vi "run_ACLooper.vi"() -> ()   [LabVIEW 2015]
uses:
  <vilib>/Platform/TimedLoop/XDataNode/timing_clust.ctl
  <vilib>/Platform/TimedLoop/XDataNode/nitl_modes.ctl
  <vilib>/Platform/TimedLoop/XDataNode/wakeup.ctl
  <vilib>/measure/matone.llb/Extract Multiple Tone Information 1 Chan.vi
  <vilib>/measure/maspectr.llb/FFT Spectrum (Mag-Phase) for 1 Chan.vi
  <vilib>/measure/matone.llb/Extract Single Tone Information 1 Chan.vi
  <vilib>/Utility/file.llb/Write To Spreadsheet File (string).vi
  <vilib>/Platform/TimedLoop/XDataNode/XDataNode.xnode
  <vilib>/Platform/TimedLoop/XDataNode/XDNodeRunTimeDep.lvlib
  <vilib>/measure/NI_MAPro.lvlib
  <vilib>/ptbypt/NI_PtbyPt.lvlib
panel:
  in  "?":T1(tab)
  in  "Number of Channel":string(combo)="2"
  in  "Volume of Sample (ml)":dbl=0.498
  in  "Concentration of Sample (mg/ml)":dbl=1.19
  in  "Select Serial Port":refnum<visa-resource-name>="COM6"
  in  "Temperature \nMeasurement":bool
  out "Value Ch4":dbl format="%.2f"
  out "Value Ch3":dbl format="%.2f"
  out "Status Ch4":bool
  out "Status Ch3":bool
  out "Status Ch2":bool
  out "Status Ch1":bool
  out "Unit Ch 4":string=" "
  out "Unit Ch 3":string=" "
  out "Value Ch2":dbl format="%.2f"
  out "Unit Ch2":string=" "
  out "Unit Ch1":string=" "
  out "Value Ch1":dbl format="%.2f"
  out "Temperature Streaming":T2(graph)={"Value_1"=28.19, "Value_2"=24.43, "Value_3"=0.0, "Value_4"=0.0}
  in  "Clear the Figure":bool
  in  "Stop":bool
  in  "Start":bool
  in  "Graph ChA":bool=TRUE
  out "Channel A":i16[](graph)
  in  "Enable ChA":bool=TRUE
  in  "Channel A Settings":T3={"Enabled"=TRUE, "DC Coupled"=TRUE, "Range"=6} {"Range" items=["10 mV", "20 mV", "50 mV", "100 mV", "200 mV", "500 mV", "1 V", "2 V", "5 V", "10 V", "20 V", "50 V ", "100 V"]}
  out "Numeric":i32
  in  "stop":bool
  in  "PicoScope":bool=TRUE
  out "Frequency Interpolate / Hz A":dbl format="%#_8g"
  out "H (A/m) / Vpp":dbl
  in  "ChA sample length":i32=5
  in  "H sample length":i32=5
  in  "Filter H":bool=TRUE
  in  "Rokoski (V(mV)/I(A))":dbl=20.0
  in  "Turns of Coil":dbl=6.0
  out "Current (A)":dbl
  in  "Filter ChA":bool=TRUE
  in  "H calculator":bool=TRUE
  out "H / Vpp":cluster{dbl}(graph)
  out "Vpp A":dbl
  out "Frequency Tracking A":cluster{"Frequency Interpolate / Hz":dbl}(graph)
  in  "Balance":bool
  in  "Description":string="no sample"
  in  "Filename":string="\\Oct04_warmup_2ch_18_4V.txt"
  in  "Time Target (min)":dbl=600.0 format="%#_13g"
  out "Measurement Complete":bool caption="Time has Elapsed"
  out "Remaining  time":dbl format="%<%H:%M:%S>t"
  in  "Record":bool
  in  "File Path":path=path "C:/Users/Fangyu/Google Drive/3_UCL MRes Medical Device/M0_Individual Project/A008 Experiments/C004_LabViewPicoScope/MACH/data"
  in  "Recording Period (ms)":i64=1000
  out "Phase (deg)":dbl format="%.2p"
  in  "MACH:":string(combo)="1. MACH/HBL Invitro 6Turn"
  out "PicoScope V range":dbl
  out "Recording Time":dbl format="%<%H:%M:%S>t"
  in  "Channel B Settings":T3={"Enabled"=TRUE, "DC Coupled"=TRUE, "Range"=7} {"Range" items=["10 mV", "20 mV", "50 mV", "100 mV", "200 mV", "500 mV", "1 V", "2 V", "5 V", "10 V", "20 V", "50 V ", "100 V"]}
  in  "Enable ChB":bool
  out "Channel B":i16[](graph)
  in  "Acquisition Settings":T4={"preTriggerSamples"=0, "postTriggerSamples"=20000, "timebase"=2, "Aggregate Data"=FALSE, "Down Sample Ratio"=1, "Four Channel Device"=FALSE, "Oversample"=1} {"Down Sample Ratio" min=1 step=1}
  in  "Sampling Frequency":dbl=250000000.0
  in  "Trigger Settings":T5={"Trigger Enabled"=TRUE, "Trigger Source"=enum."Channel A", "Trigger Threshold (16-bit counts)"=100, "Trigger Direction"=3, "Trigger Delay (samples)"=20, "Auto Trigger Time (ms)"=0} {"Trigger Direction" items=["Rising"=2, "Falling"=3]}
  in  "History data for graph reset":cluster{dbl}[](array[cluster])
  in  "Calibration":bool
  in  "Commands":string
  in  "Send/Enter:":bool
  in  "Slect Probet Channel":string="1,3"
  in  "Send/Enter: 2":bool
  in  "Reset":bool
  in  "Check Param":bool
  out "read buffer":string="PS??\r\nPS??\r\nAE??\r\n\n <ignored>\r\nPS=1,2\r\n"
  out "error out 2":errorcluster={"status"=TRUE, "code"=-1073807339, "source"="VISA Read in Test1.vi"}
  # "Setting of Luxtron Thermometer"
  # "1.  Enter Cal Temperature in 'Commands' above\n     (CT=XX.X)  and press 'Send' button\n2.  Press button below\n3.  Calibration may take ~ 1 min."
  # "The content of recorded data:\n1st Row; 2nd Row; 3rd Row; 4th Row; 5th Row; 6th Row; 7th Row; 8th Row; 9th Row\nTime; Field Strength; Frequency; Value Ch1; Value Ch2; Value Ch3; Value Ch4; Maximal Frequency; ;Frequency Drop"
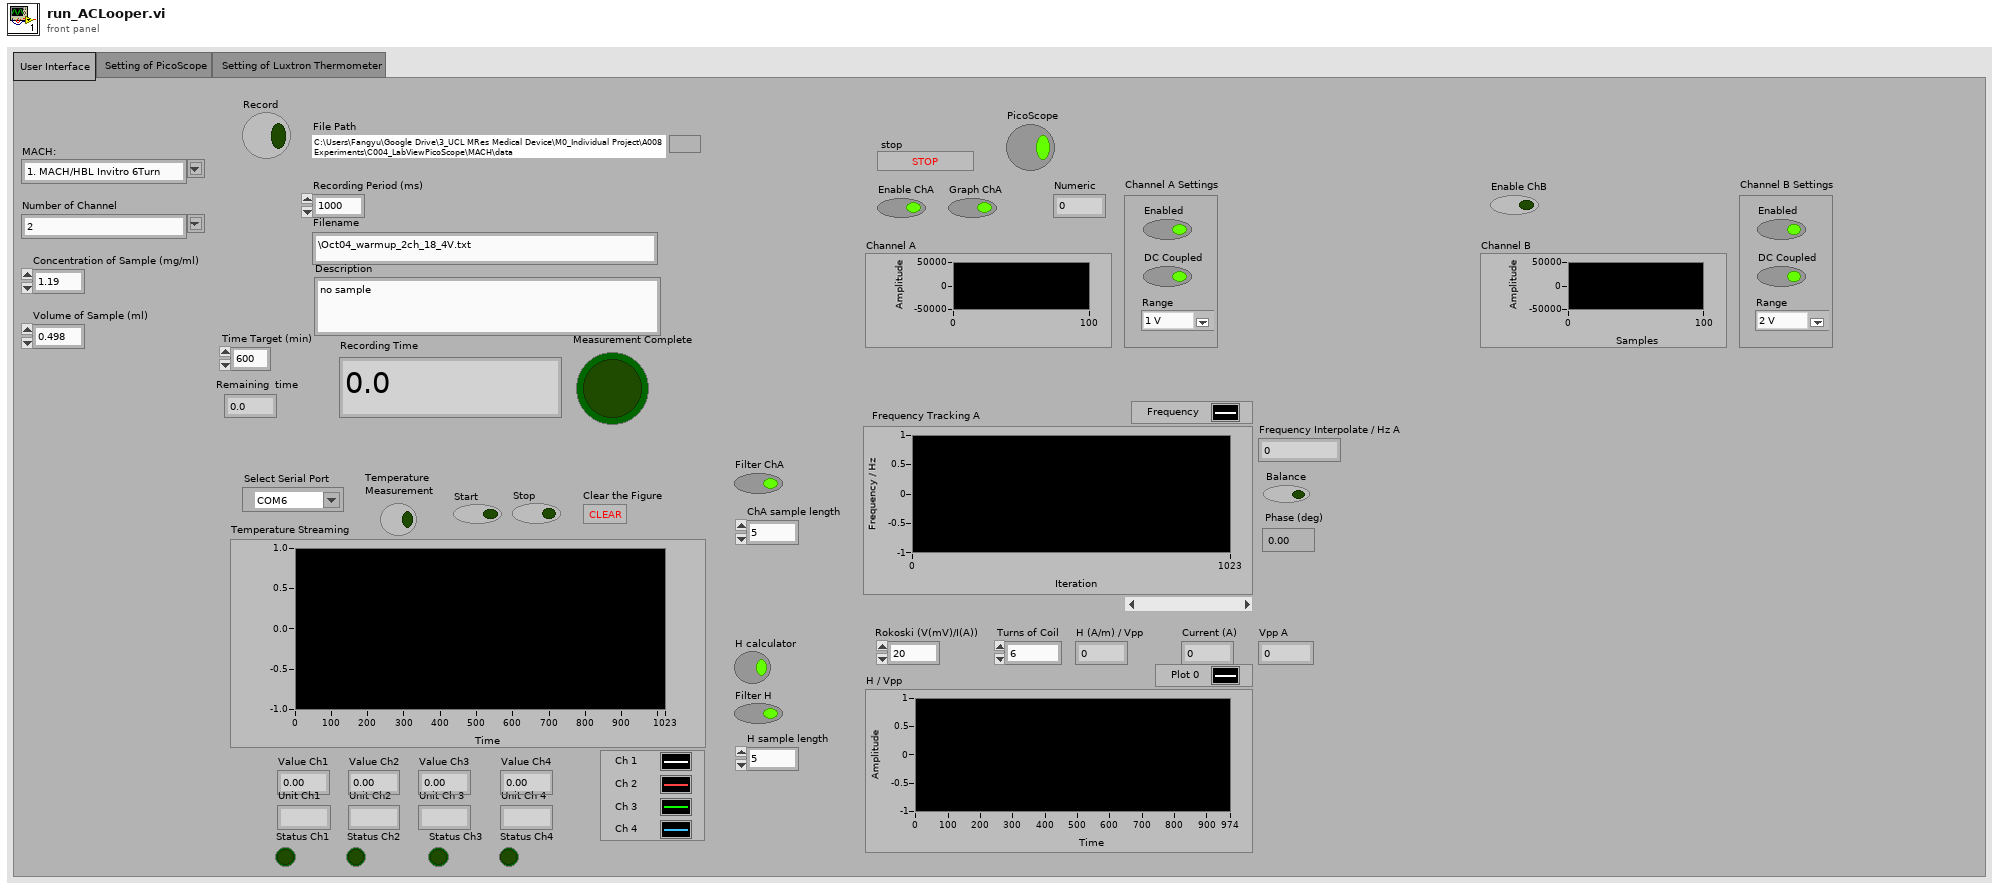
[diagram p1: front panel]
types:
  T1 = enum32{"User Interface", " Setting of PicoScope", " Setting of Luxtron Thermometer"}
  T2 = cluster{"Value_1":dbl, "Value_2":dbl, "Value_3":dbl, "Value_4":dbl}
  T3 = cluster{"Enabled":bool, "DC Coupled":bool, "Range":u16}
  T4 = cluster{"preTriggerSamples":i32, "postTriggerSamples":i32, "timebase":u32, "Aggregate Data":bool, "Down Sample Ratio":u32, "Four Channel Device":bool, "Oversample":i16}
  T5 = cluster{"Trigger Enabled":bool, "Trigger Source":enum16{"Channel A", "Channel B", "Channel C", "Channel D"}, "Trigger Threshold (16-bit counts)":i16, "Trigger Direction":u16, "Trigger Delay (samples)":u32, "Auto Trigger Time (ms)":i16}
  T6 = cluster{"Status_1":bool, "Value_1":dbl, "Unit_1":string, "Status_2":bool, "Value_2":dbl, "Unit_2":string, "Status_3":bool, "Value_3":dbl, "Unit_3":string, "Status_4":bool, "Value_4":dbl, "Unit_4":string}
  T7 = enum32{"none", "input signal", "detected signal", "residual signal"}
  T8 = cluster{"Peak-to-Peak Voltage (microvolts)":u32, "Offset Voltage (microvolts)":i32, "Wave Type":i16, "Sweep Type":i32, "Shots":u32, "Sweeps":u32, "Trigger Type":i32, "Trigger Source":i32, "Ext. Threshold (ADC count)":i16, "White Noise":bool}
  T9 = cluster{"Channel D Buffer":i16[], "Channel C Buffer":i16[], "Channel B Buffer":i16[], "Channel A Buffer":i16[]}
  T10 = cluster{"detected frequency":dbl, "detected amplitude":dbl, "detected phase (deg)":dbl}[]
  T11 = cluster{"magnitude[0]":dbl, "magnitude[1]":dbl, "magnitude[2]":dbl, "magnitude[3]":dbl, "magnitude[4]":dbl, "magnitude[5]":dbl, "magnitude[6]":dbl, "magnitude[7]":dbl, "magnitude[8]":dbl}
  T12 = typedef "XDNodeRunTimeDep.lvlib/timing_clust.ctl" = cluster{"Expected End [f-1]":u64, "Actual End [f-1]":u64, "Finished Late? [f-1]":bool, "Expected End [i-1]":u64, "Actual End [i-1]":u64, "Finished Late? [i-1]":bool, "Expected Start [i]":u64, "Actual Start [i]":u64, "Expected Start [f]":u64, "Actual Start [f]":u64, "Source Name":string, "Structure Name":string, "Period":i64, "Deadline":i64, "Offset":i64, "Start":i64, "Priority":i32, "Timeout":i32, "Mode":T13, "Wakeup Reason":T14, "Error":errorcluster, "Source Type":string, "Secondary Source Type":string, "Global End Time":u64, "Global Start Time":u64, "Frame Duration":u64, "Iteration Duration":u64, "Assigned CPU":i32, "I/O Scan Engine Mode":u32}
  T13 = typedef "XDNodeRunTimeDep.lvlib/nitl_modes.ctl" = enum32{"No Change", "Process missed periods, maintain original phase", "Discard missed periods, maintain original phase", "Process missed periods, ignore original phase", "Discard missed periods, ignore original phase"}
  T14 = typedef "XDNodeRunTimeDep.lvlib/wakeup.ctl" = enum32{"Normal", "Aborted", "Asynchronous wakeup", "Timing source error", "Timed loop error", "Timeout"}
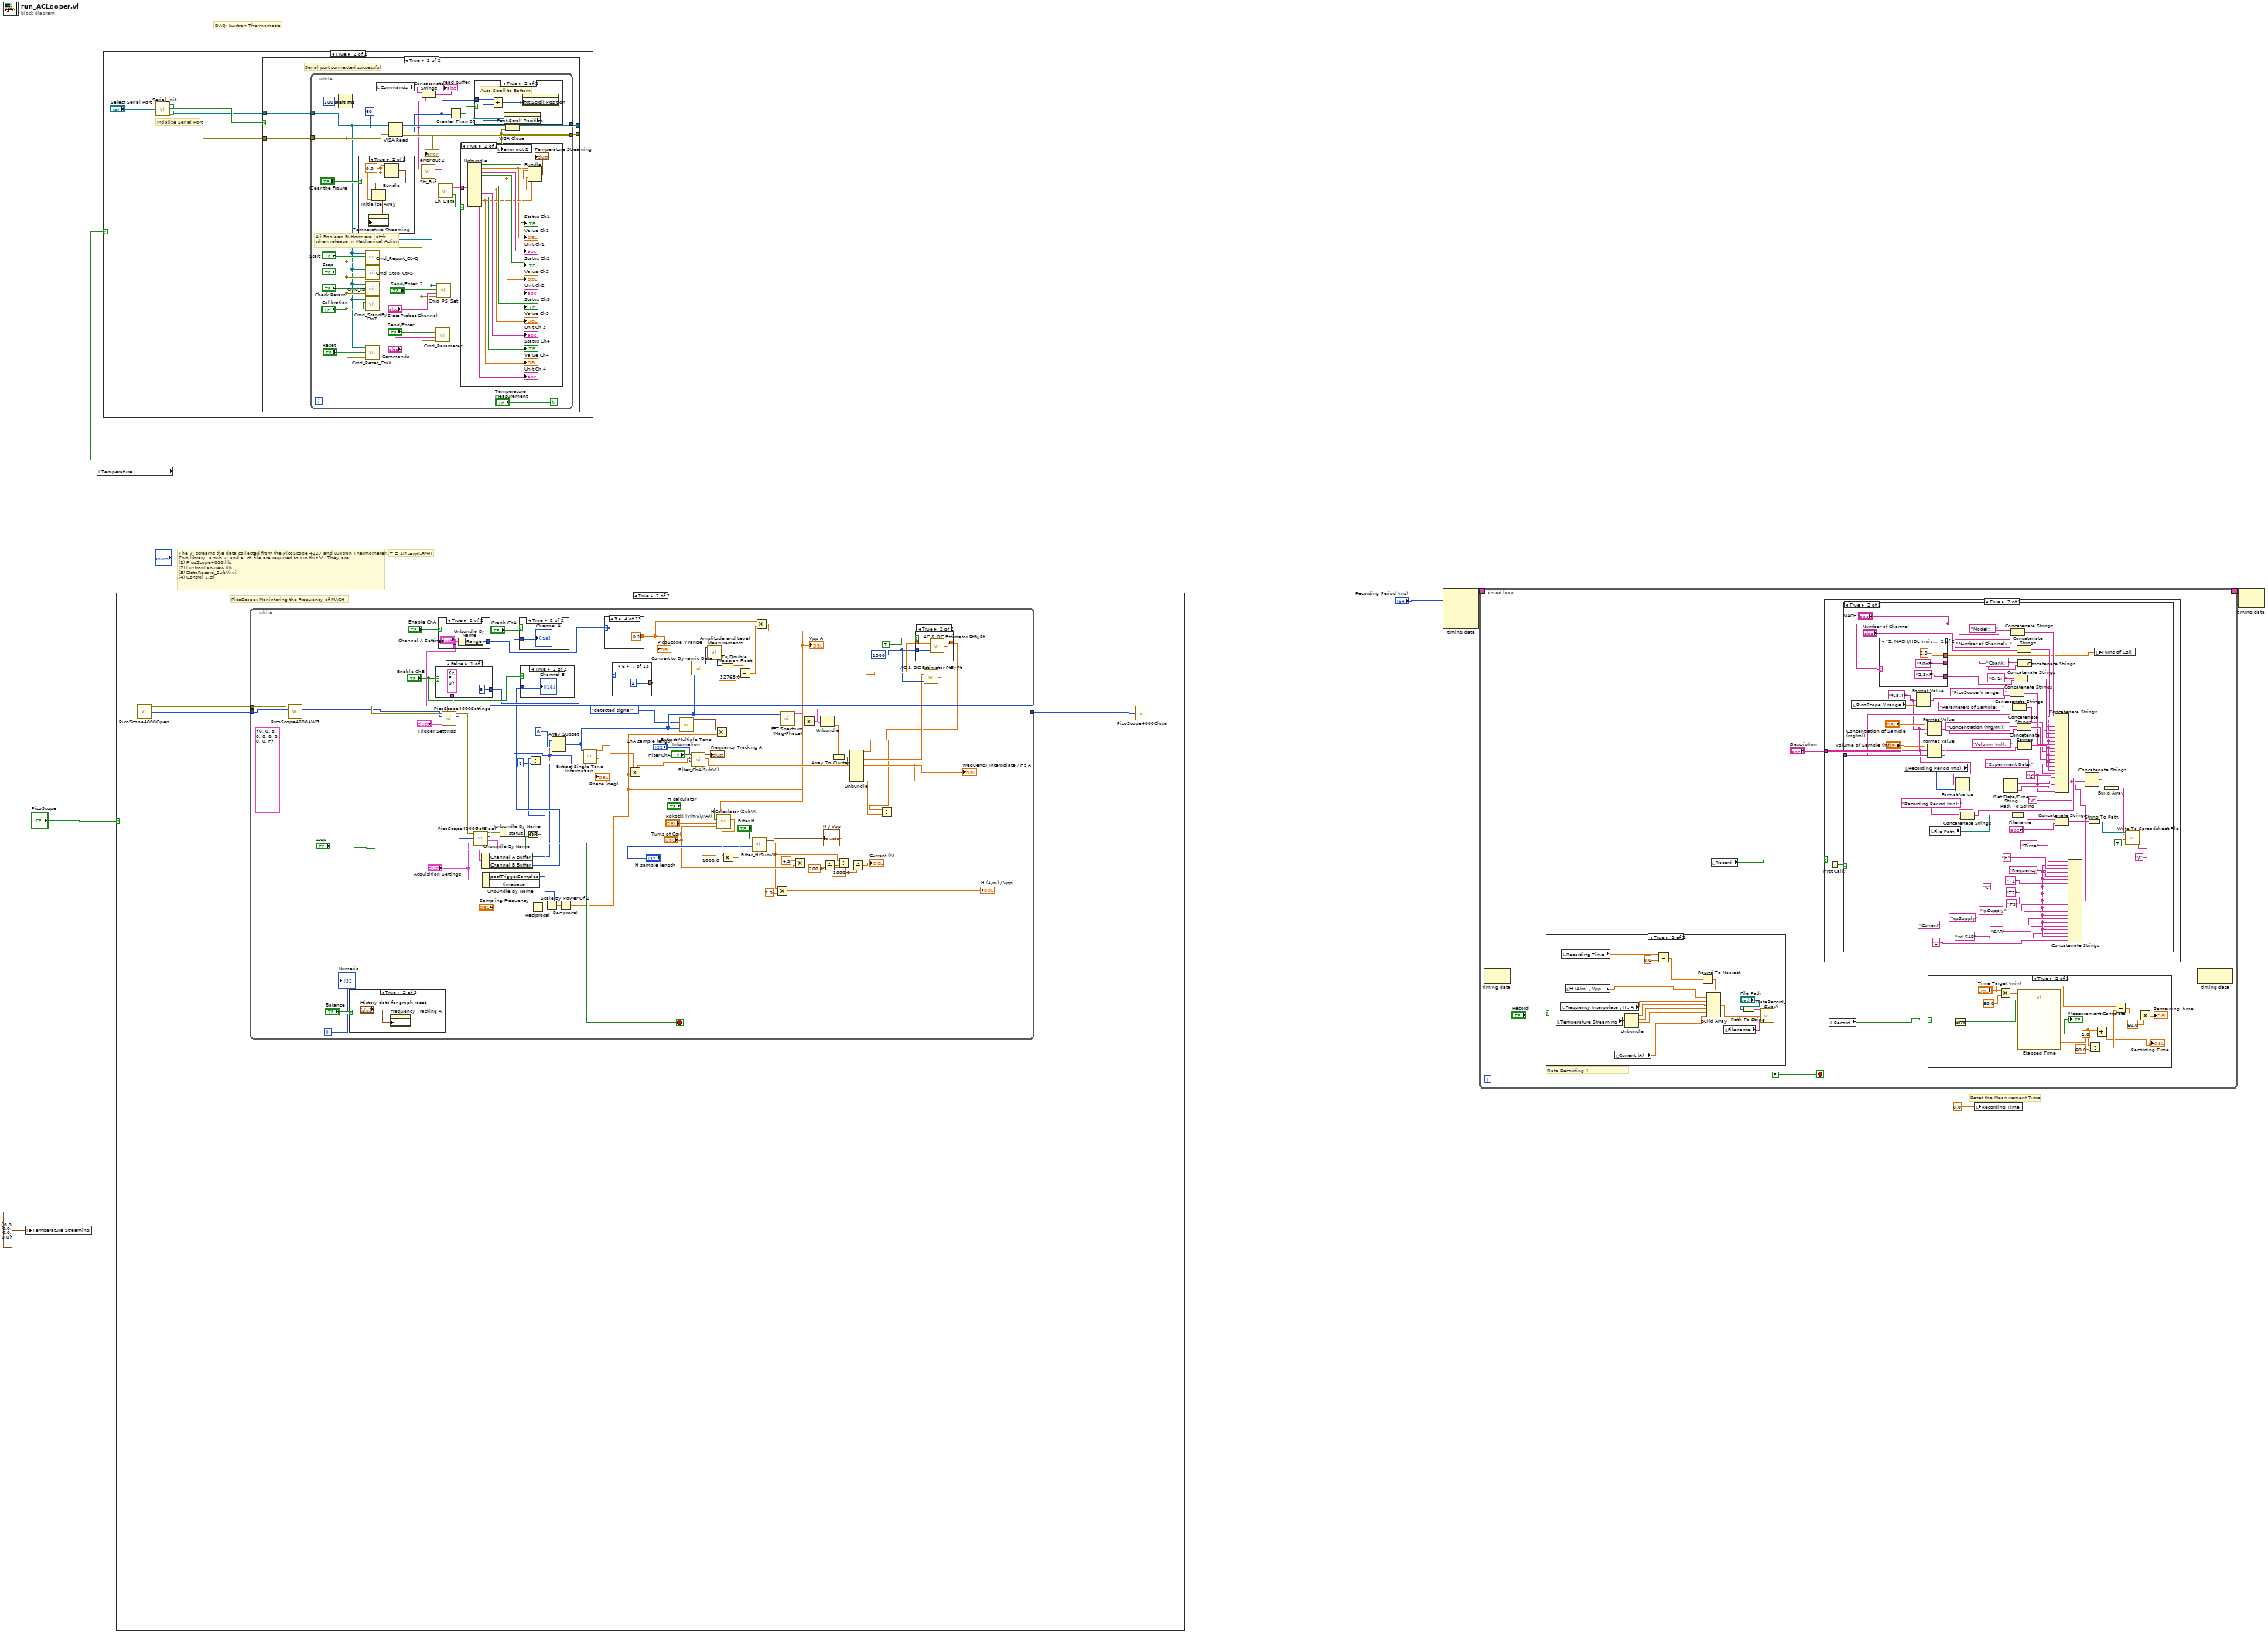
[diagram p0: block diagram]
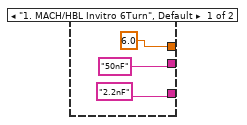
[diagram p4: hidden frame]
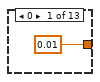
[diagram p9: hidden frame]
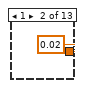
[diagram p10: hidden frame]
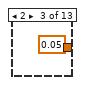
[diagram p11: hidden frame]
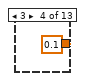
[diagram p12: hidden frame]
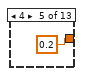
[diagram p13: hidden frame]
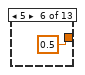
[diagram p14: hidden frame]
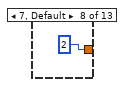
[diagram p15: hidden frame]
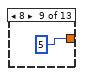
[diagram p16: hidden frame]
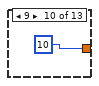
[diagram p17: hidden frame]
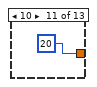
[diagram p18: hidden frame]
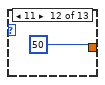
[diagram p19: hidden frame]
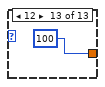
[diagram p20: hidden frame]
diagram:
  # "Reset the Measurement Time"
  # "T = A(1-exp(-B*t))"
  # "The vi screams the data collected from the PicoScope 4227 and Luxtron Thermometer. \nTwo library, a sub vi and a .ctl file are required to run this Vi. They are:\n(1) PicoScope4000.llb\n(2) LuxtronLabview.llb\n(3) DataRecord_SubVi.vi\n(4) Control 1.ctl"
  # "DAQ: Luxtron Thermometre"
  n1 = local write "Temperature Streaming"(T2 {"Value_1"=0.0, "Value_2"=0.0, "Value_3"=0.0, "Value_4"=0.0} ("Temperature Streaming")) -> ()
  n2 = local read "Temperature \nMeasurement"() -> (w7:bool)
  n3 = case shown="True" w7 {
    frame False {
    }
    frame True {
      # "Intialize Serial Port"
      n4 = call "Serial_init.vi"("VISA resource name"="Select Serial Port") -> ("duplicate VISA resource name"=w9:refnum<visa-resource-name>, "Open Successully"=w10:bool, "error out"=w11:errorcluster)
      n5 = case shown="True" w10 {
        tunnel: w11 -> [w15 w18]
        tunnel: [w15 w19] -> w13
        tunnel: w9 -> [w14 w17]
        tunnel: [w14 w16] -> w8
        frame False {
        }
        frame True {
          # "Serial port connected successful"
          n6 = while {
            tunnel: [w42] -> w19
            tunnel: [w44] -> w16
            tunnel: w18 -> [w24]
            tunnel: w17 -> [w23]
            stop <- "Temperature \nMeasurement" continue-if-true
            # "All Boolean Buttons are Latch\nwhen release in Mechanical Action"
            n7 = Wait (ms)(milliseconds to wait=u32 100 ("millisecond multiple")) -> ()  [unwired: 1 out]
            n8 = case shown="True" "Clear the Figure" {
              frame False {
              }
              frame True {
                w63 = 0.0
                n9 = Bundle(w63, w63, w63, w63) -> (w64:cluster{dbl, dbl, dbl, dbl})  [unwired: 1 in]
                n10 = Initialize Array(w64, w63) -> (w62:cluster{dbl, dbl, dbl, dbl}[])
                n11 = property on="Temperature Streaming" class="WFChart (strict)"("History Data"=w62) -> ()  [unwired: 2 in, 2 out]
              }
            }
            n12 = call "Cmd_Report_Ctr-Q.vi"("error IN"=w24, "Send Report Cmd"="Start", "duplicate VISA resource name"=w23) -> ()  [unwired: 2 out]
            n13 = call "Cmd_Stop_Ctr-S.vi"("error in"=w24, "Send Report Cmd"="Stop", "duplicate VISA resource name"=w23) -> ()  [unwired: 2 out]
            n14 = call "Cmd_ID.vi"("error IN"=w24, "Send Report Cmd"="Check Param", "duplicate VISA resource name"=w23) -> ()  [unwired: 2 out]
            n15 = call "Cmd_StandBy_Ctr-T.vi"("error IN"=w24, "Send Report Cmd"="Calibration", "duplicate VISA resource name"=w23) -> ()  [unwired: 2 out]
            n16 = call "Cmd_Reset_Ctr-X.vi"("error IN"=w24, "Send Report Cmd"="Reset", "duplicate VISA resource name"=w23) -> ()  [unwired: 2 out]
            n17 = local read "Commands"() -> (w21:string)
            n18 = VISA Read(VISA resource name=w23, byte count=u32 60 ("byte count (0)"), error in (no error)=w24) -> (VISA resource name out=w44:refnum<visa-resource-name>, read buffer=w33:string, return count=w34:u32, error out=w42:errorcluster)
            "error out 2" <- w42
            n19 = call "Str_Buf.vi"("String_in"=w33) -> ("String_Out"=w31:string)  [unwired: 3 out]
            n20 = Concatenate Strings(w21, w33) -> (→"read buffer":string)
            n21 = call "Cmd_Parameter.vi"("error IN"=w24, "Command & Parameter"="Commands", "Send Command"="Send/Enter:", "duplicate VISA resource name"=w23) -> ()  [unwired: 2 out]
            n22 = call "Cmd_PS_Set.vi"("error IN"=w24, "Write String"="Slect Probet Channel", "Send Command"="Send/Enter: 2", "duplicate VISA resource name"=w23) -> ()  [unwired: 2 out]
            n23 = call "Ch_Data.vi"("String"=w31) -> ("output cluster"=w32:T6, "FormatOK"=w30:bool)
            n24 = Greater Than 0?(x=w34) -> (x > 0?=w35:bool)
            n25 = case shown="True" w30 {
              tunnel: w32 -> [_ w48]
              frame False {
              }
              frame True {
                n26 = Unbundle(w48) -> ("Status_1"=→"Status Ch1":bool, "Value_1"=w47:dbl, "Unit_1"=→"Unit Ch1":string, "Status_2"=→"Status Ch2":bool, "Value_2"=w46:dbl, "Unit_2"=→"Unit Ch2":string, "Status_3"=→"Status Ch3":bool, "Value_3"=w45:dbl, "Unit_3"=→"Unit Ch 3":string, "Status_4"=→"Status Ch4":bool, "Value_4"=w50:dbl, "Unit_4"=→"Unit Ch 4":string)
                "Value Ch1" <- w47
                "Value Ch2" <- w46
                "Value Ch3" <- w45
                "Value Ch4" <- w50
                n27 = Bundle("Value_1"=w47, "Value_2"=w46, "Value_3"=w45, "Value_4"=w50) -> (→"Temperature Streaming":T2)  [unwired: 1 in]
              }
            }
            n28 = case shown="True" w35 {
              tunnel: w34 -> [_ w60]
              frame False {
              }
              frame True {
                # "Auto Scroll to Bottom"
                n29 = property class="Str"() -> ("Text.Scroll Position"=w59:u32)  [unwired: 2 in, 2 out]
                n30 = Add(x=w60, y=w59) -> (x+y=w61:u32)
                n31 = property class="Str"("Text.Scroll Position"=w61) -> ()  [unwired: 2 in, 2 out]
              }
            }
          }
        }
      }
      n32 = local write "error out 2"(w13) -> ()
      n33 = VISA Close(VISA resource name=w8, error in (no error)=w13) -> ()  [unwired: 1 out]
    }
  }
  n34 = case shown="True" "PicoScope" {
    frame False {
    }
    frame True {
      # "PicoScope: Monintoring the Frequency of MACH"
      n35 = call "PicoScope4000Open.vi"() -> ("error out"=w67:errorcluster, "handle"=w65:i16)  [unwired: 1 in, 1 out]
      n36 = while {
        tunnel: w67 -> [w144]
        tunnel: [w146] -> w66
        tunnel: w65 -> [w143]
        i -> [w145]
        stop <- w140 stop-if-true
        w77 = 1000 ("sample length")
        (unwired) T8 {"Peak-to-Peak Voltage (microvolts)"=0, "Offset Voltage (microvolts)"=0, "Wave Type"=8, "Sweep Type"=0, "Shots"=0, "Sweeps"=0, "Trigger Type"=0, "Trigger Source"=0, "Ext. Threshold (ADC count)"=0, "White Noise"=FALSE} ("General AWG Settings")
        n37 = call "PicoScope4000AWG.vi"("Handle In"=w143, "error in"=w144) -> ("Handle Out"=w141:i16, "error out"=w142:errorcluster)  [unwired: 8 in]
        n38 = case shown="True" "Balance" {
          frame False {
          }
          frame True {
            n39 = property on="Frequency Tracking A" class="WFChart (strict)"("History Data"="History data for graph reset") -> ()  [unwired: 2 in, 2 out]
          }
        }
        n40 = case shown="False" "Enable ChB" {
          tunnel: [T3 {"Enabled"=FALSE, "DC Coupled"=FALSE, "Range"=0} ("Channel A Settings") "Channel B Settings"] -> w124
          tunnel: [u16 6 ("Range") w182] -> w116
          frame False {
          }
          frame True {
            n41 = Unbundle By Name("Channel B Settings") -> ("Range"=w182:u16)
          }
        }
        n42 = case shown="True" "Enable ChA" {
          tunnel: [T3 {"Enabled"=FALSE, "DC Coupled"=FALSE, "Range"=0} ("Channel A Settings") "Channel A Settings"] -> w123
          tunnel: [u16 6 ("Range") w186] -> w117
          frame False {
          }
          frame True {
            n43 = Unbundle By Name("Channel A Settings") -> ("Range"=w186:u16)
          }
        }
        n44 = call "PicoScope4000Settings.vi"("Channel B Settings"=w124, "Channel A Settings"=w123, "Trigger Settings"="Trigger Settings", "handle in"=w141, "error in"=w142) -> ("handle out"=w129:i16, "error out"=w128:errorcluster)  [unwired: 5 in]
        n45 = call "PicoScope4000GetBlock.vi"("error in"=w128, "handle in"=w129, "Acquisition Settings"="Acquisition Settings") -> ("error out"=w136:errorcluster, "handle out"=w146:i16, "Buffers (Max or non-aggregated)"=w135:T9)  [unwired: 3 in, 2 out]
        n46 = Unbundle By Name(w135) -> ("Channel A Buffer"=w96:i16[], "Channel B Buffer"=w115:i16[])
        n47 = Unbundle By Name("Acquisition Settings") -> ("postTriggerSamples"=w100:i32, "timebase"=w130:u32)
        n48 = Unbundle By Name(w136) -> ("status"=w134:bool)
        n49 = case shown="True" "Graph ChA" {
          tunnel: w96 -> [_ w179]
          frame False {
          }
          frame True {
            "Channel A" <- w179
          }
        }
        n50 = case shown="True" "Enable ChB" {
          tunnel: w115 -> [_ w178]
          frame False {
          }
          frame True {
            "Channel B" <- w178
          }
        }
        n51 = Or(x=w134, y="stop") -> (x .or. y?=w140:bool)
        n52 = Divide(x=w100, y=1) -> (x/y=w98:dbl)
        n53 = Reciprocal(x="Sampling Frequency") -> (1/x=w132:dbl)
        n54 = Scale By Power Of 2(n=w130, x=w132) -> (x*2^n=w131:dbl)
        n55 = Array Subset(array=w96, index=0, length=w98) -> (w73:i16[])
        n56 = Reciprocal(x=w131) -> (1/x=w68:dbl)
        n57 = call-poly <vilib>:"Extract Single Tone Information.vi"("time signal in"=w73) -> ("detected phase (deg)"=→"Phase (deg)":dbl, "detected frequency"=w108:dbl)  [unwired: 5 in, 4 out]
        n58 = case shown="3" w117 {
          tunnel: [0.01 0.02 0.05 0.1 0.2 0.5 1 2 5 10 20 50 100] -> w107
          frame 0 {
          }
          frame 1 {
          }
          frame 2 {
          }
          frame 3 {
          }
          frame 4 {
          }
          frame 5 {
          }
          frame 6 {
          }
          frame 7, Default {
          }
          frame 8 {
          }
          frame 9 {
          }
          frame 10 {
          }
          frame 11 {
          }
          frame 12 {
          }
        }
        "PicoScope V range" <- w107
        n59 = case shown="6" w116 {
          tunnel: [0.01 0.02 0.05 0.1 0.2 0.5 1 2 5 10 20 50 100] -> _
          frame 0 {
          }
          frame 1 {
          }
          frame 2 {
          }
          frame 3 {
          }
          frame 4 {
          }
          frame 5 {
          }
          frame 6 {
          }
          frame 7, Default {
          }
          frame 8 {
          }
          frame 9 {
          }
          frame 10 {
          }
          frame 11 {
          }
          frame 12 {
          }
        }
        n60 = Multiply(x=w108, y=w68) -> (x*y=w109:dbl)
        n61 = call-poly <vilib>:"Extract Multiple Tone Information.vi"("time signal in"=w73, "export mode"=T7."detected signal") -> ("multiple tone information"=w72:T10)  [unwired: 11 in, 2 out]
        n62 = call "Convert to Dynamic Data"("Array"=w73) -> ("Dynamic Data Type"=w104:dynamicdata)  [unwired: 3 in]
        n63 = call "Filter_ChA(SubVI).vi"("sample length"="ChA sample length", "input"=w109, "Filter on"="Filter ChA") -> ("Output Number"=→"Frequency Interpolate / Hz A":dbl, "Output"=→"Frequency Tracking A":cluster{"Frequency Interpolate / Hz":dbl})  [unwired: 7 in]
        n64 = call "Amplitude and Level Measurements"("Signals"=w104) -> ("Peak to Peak"=w94:dynamicdata)  [unwired: 13 in, 1 out]
        n65 = Multiply(x=w72, y=w68) -> ()  [unwired: 1 out]
        n66 = To Double Precision Float(number=w94) -> (double precision float=w93:dbl)
        n67 = Divide(x=w93, y=32768.0) -> (x/y=w103:dbl)
        n68 = Multiply(x=w107, y=w103) -> (x*y=w102:dbl)
        "Vpp A" <- w102
        n69 = call "HCalculator (SubVI).vi"("Turns of Coil"="Turns of Coil", "Rokoski (V(mV)/I(A))"="Rokoski (V(mV)/I(A))", "H calculator"="H calculator", "Vpp in"=w102) -> ("Vpp out"=w112:dbl)  [unwired: 6 in, 1 out]
        n70 = Multiply(x=w112, y=1000.0) -> (x*y=w111:dbl)
        n71 = call "Filter_H(SubVI).vi"("sample length"="H sample length", "input"=w111, "Filter on"="Filter H") -> ("Output Number"=w86:dbl, "Output"=→"H / Vpp":cluster{"Frequency Interpolate / Hz":dbl})  [unwired: 7 in]
        n72 = Multiply(x=w86, y=1.0) -> (x*y=→"H (A/m) / Vpp":dbl)
        n73 = call-poly <vilib>:"FFT Spectrum (Mag-Phase).vi"("time signal"=w73) -> ("magnitude"=w69:cluster{"f0":dbl, "df":dbl, "magnitude":dbl[]})  [unwired: 6 in, 4 out]
        n74 = Multiply(x=4.5, y="Turns of Coil") -> (x*y=w89:dbl)
        n75 = Multiply(x=w69, y=w68) -> (x*y=w70:cluster{"f0":dbl, "df":dbl, "magnitude":dbl[]})
        n76 = Unbundle(w70) -> ("magnitude"=w81:dbl[])  [unwired: 2 out]
        n77 = Divide(x=w89, y=200.0) -> (x/y=w87:dbl)
        n78 = Array To Cluster(array=w81) -> (cluster=w80:T11)
        n79 = Divide(x=w86, y=w87) -> (x/y=w85:dbl)
        n80 = Unbundle(w80) -> ("magnitude[0]"=w78:dbl, "magnitude[2]"=w76:dbl)  [unwired: 7 out]
        n81 = Divide(x=w85, y=1000.0) -> (x/y=→"Current (A)":dbl)
        n82 = case shown="True" TRUE ("Filter on") {
          tunnel: w78 -> [w148 w151]
          tunnel: [w148 w150] -> w75
          tunnel: w77 -> [_ w149]
          frame False {
          }
          frame True {
            n83 = call <vilib>:"AC & DC Estimator PtByPt.vi"("signal"=w151, "sample length"=w149) -> ("DC estimate (V)"=w150:dbl)  [unwired: 1 in, 2 out]
          }
        }
        n84 = call <vilib>:"AC & DC Estimator PtByPt.vi"("signal"=w76, "sample length"=w77) -> ("DC estimate (V)"=w74:dbl)  [unwired: 1 in, 2 out]
        n85 = Divide(x=w75, y=w74) -> ()  [unwired: 1 out]
        "Numeric" <- w145
      }
      n86 = call "PicoScope4000Close.vi"("handle"=w66) -> ()
    }
  }
  n87 = node-c288("Recording Period (ms)") -> (w5:T12)  [unwired: 3 in]
  n88 = timed-loop {
    timing: w5 -> [_]
    timing-out: [_] -> w4
    stop <- FALSE stop-if-true
    # "Data Recording 1"
    n89 = node-c288() -> ()  [unwired: 1 in, 1 out]
    n90 = case shown="True" "Record" {
      frame False {
      }
      frame True {
        n91 = local read "Temperature Streaming"() -> (w294:T2)
        n92 = local read "Frequency Interpolate / Hz A"() -> (w290:dbl)
        n93 = local read "Recording Time"() -> (w283:dbl)
        n94 = local read "H (A/m) / Vpp"() -> (w285:dbl)
        n95 = local read "Current (A)"() -> (w281:dbl)
        n96 = Unbundle(w294) -> ("Value_1"=w289:dbl, "Value_2"=w288:dbl, "Value_3"=w287:dbl)  [unwired: 1 out]
        n97 = Subtract(x=w283, y=0.0) -> (x-y=w282:dbl)
        n98 = Round To Nearest(number=w282) -> (nearest integer value=w284:dbl)
        n99 = Build Array(w284, w285, w290, w289, w288, w287, w281) -> (w293:dbl[])
        n100 = local read "Filename"() -> (w286:string)
        n101 = Path To String(path="File Path") -> (string=w292:string)
        n102 = call "DataRecord_SubVi.vi"("string"=w286, "Array"=w293, "File Path"=w292) -> ()
      }
    }
    n103 = local read "Record"() -> (w190:bool)
    n104 = case shown="True" w190 {
      tunnel: "Description" -> [_ w194]
      frame False {
      }
      frame True {
        n105 = First Call?() -> (First Call?: T/F=w195:bool)
        n106 = case shown="True" w195 {
          tunnel: w194 -> [_ w206]
          frame False {
          }
          frame True {
            w201 = "%5.4f" ("format string")
            w209 = "\r"
            w199 = "\t"
            w241 = "\t"
            n107 = local read "PicoScope V range"() -> (w205:dbl)
            n108 = case shown="\"2. MACH/HBL Invivo A\"" "MACH:" {
              tunnel: ["50nF" ("element") "50nF" ("element")] -> w215
              tunnel: ["2.2nF" ("element") "2.3nF" ("element")] -> w214
              tunnel: [6.0 ("Turns of Coil") 2.0 ("Turns of Coil")] -> w211
              frame "1. MACH/HBL Invitro 6Turn", Default {
              }
              frame "2. MACH/HBL Invivo A" {
              }
            }
            n109 = local read "Recording Period (ms)"() -> (w202:i64)
            n110 = Format Value(format string=w201, value (0)=w205) -> (output string=w212:string)  [unwired: 1 in]
            n111 = Format Value(format string=w201, value (0)="Concentration of Sample (mg/ml)") -> (output string=w217:string)  [unwired: 1 in]
            n112 = Format Value(format string=w201, value (0)="Volume of Sample (ml)") -> (output string=w216:string)  [unwired: 1 in]
            n113 = local read "File Path"() -> (w238:path)
            n114 = Format Value(format string=w201, value (0)=w202) -> (output string=w234:string)  [unwired: 1 in]
            n115 = Concatenate Strings("Recording Period (ms): " ("string"), w234) -> (w235:string)
            n116 = Get Date/Time String() -> (date string=w252:string, time string=w251:string)  [unwired: 3 in]
            n117 = Concatenate Strings("PicoScope V range:   " ("element"), w212) -> (w222:string)
            n118 = Path To String(path=w238) -> (string=w239:string)
            n119 = Concatenate Strings("Model:    " ("element"), "MACH:") -> (w218:string)
            n120 = Concatenate Strings("Parameters of Sample:   " ("element"), w206) -> (w208:string)
            n121 = Concatenate Strings("Cx1:  " ("element"), w214) -> (w221:string)
            n122 = Concatenate Strings("Number of Channel:  " ("element"), "Number of Channel") -> (w219:string)
            n123 = Concatenate Strings("Concentration (mg/ml):   " ("element"), w217) -> (w223:string)
            n124 = Concatenate Strings("Cbank:  " ("element"), w215) -> (w220:string)
            n125 = Concatenate Strings("Volumn (ml):   " ("element"), w216) -> (w224:string)
            n126 = Concatenate Strings(w218, w209, w219, w209, w220, w209, w221, w209, w222, w209, w208, w209, w223, w209, w224, w209, "Experiment Date:" ("element"), w241, w252, w241, w251, w241) -> (w236:string)
            n127 = Concatenate Strings(w239, "Filename") -> (w255:string)
            n128 = Concatenate Strings("Time" ("string"), w199, "H" ("string"), w199, "Frequency" ("string"), w199, "T1" ("string"), w199, "T2" ("string"), w199, "T3" ("string"), w199, "IpSupply" ("string"), w199, "VpSupply" ("string"), w199, "Current" ("string"), w199, "SAR" ("string"), w199, "sd SAR" ("string"), w199, "L" ("string")) -> (w237:string)
            n129 = Concatenate Strings(w236, w235, w209, w237) -> (w243:string)
            n130 = String To Path(string=w255) -> (path=w254:path)
            n131 = local write "Turns of Coil"(w211) -> ()
            n132 = Build Array(w243) -> (w250:string[])
            n133 = call-poly <vilib>:"Write To Spreadsheet File.vi"("delimiter (\\t)"="\t", "append to file? (new file:F)"=TRUE, "1D data"=w250, "file path (dialog if empty)"=w254) -> ()  [unwired: 4 in, 1 out]
          }
        }
      }
    }
    n134 = local read "Record"() -> (w189:bool)
    n135 = case shown="True" w189 {
      selector: w189 -> [_ w269]
      frame False {
      }
      frame True {
        n136 = Not(x=w269) -> (.not. x?=w268:bool)
        n137 = Multiply(x="Time Target (min)", y=60.0) -> (x*y=w276:dbl)
        n138 = call "Elapsed Time"("Time Target (s)"=w276, "Reset"=w268) -> ("Elapsed Time (s)"=w266:dbl, "Time has Elapsed"=→"Measurement Complete":bool)  [unwired: 10 in, 6 out]
        n139 = Divide(x=w266, y=60.0) -> (x/y=w270:dbl)
        n140 = Add(x=w266, y=1.0) -> (x+y=→"Recording Time":dbl)
        n141 = Subtract(x="Time Target (min)", y=w270) -> (x-y=w273:dbl)
        n142 = Multiply(x=w273, y=60.0) -> (x*y=→"Remaining  time":dbl)
      }
    }
    n143 = node-c288() -> ()  [unwired: 1 in, 1 out]
  }
  n144 = local write "Recording Time"(0.0 ("Measurement Time")) -> ()
  n145 = node-c288(w4) -> ()  [unwired: 1 out]
